vi "get error contents.vi"(9 "Variables in":T1, 11 "New errors":refnum<class "Incident.lvclass">[](array[class])) -> (1 "Variables out":T1, 3 "table string":string[][](array[string]))   [LabVIEW 2018]
uses:
  type defs/Comms loop variables.ctl
  Chris VIs/Incident logger/Incidents/Incident.lvclass
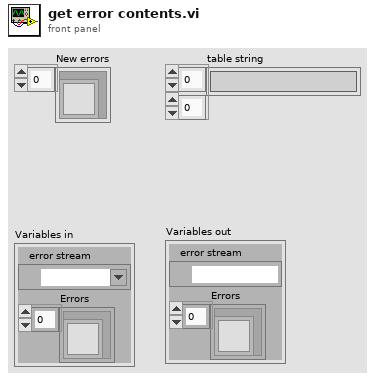
[diagram p1: front panel]
types:
  T1 = typedef "Comms loop variables.ctl" = cluster{"error stream":refnum<k21>, "Errors":refnum<class "Incident.lvclass">[]}
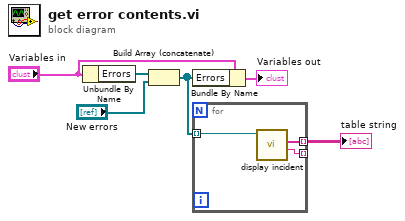
[diagram p0: block diagram]
diagram:
  n1 = Unbundle By Name("Variables in") -> ("Errors"=w4:refnum<class "Incident.lvclass">[])
  n2 = Build Array (concatenate)(w4, "New errors") -> (w2:refnum<class "Incident.lvclass">[])
  n3 = Bundle By Name(cluster="Variables in", "Errors"=w2) -> (→"Variables out":T1)
  n4 = for {
    tunnel: w2 -> [w9] mode=indexing
    tunnel: [w8] -> w6 mode=indexing
    tunnel: [w7] -> _ mode=indexing
    n5 = call-dynamic "display incident.vi"("Incident in"=w9) -> ("Incident type"=w7:string, "table string"=w8:string[])  [unwired: 5 in, 4 out]
  }
  "table string" <- w6
